vi "gRPC OOB Comm.vi"(6 "Main to gRPC":T2, 11 "Node in":refnum<class "ThermotronDriver.lvclass">) -> (1 "Update gRPC":bool, 3 "Node out":refnum<class "ThermotronDriver.lvclass">, 4 "gRPC to Main":T1)   [LabVIEW 2023, in "ThermotronDriver.lvlib" / "ThermotronDriver.lvclass"]
uses:
  ThermotronDriver.lvclass
  Type Defs/Main to gRPC.ctl
  Type Defs/gRPC to Main.ctl
  ThermotronDriver.lvclass/ThermotronDriver.ctl
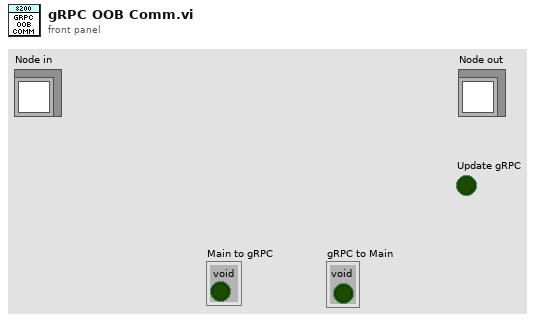
[diagram p1: front panel]
types:
  T1 = typedef "ThermotronDriver.lvlib/ThermotronDriver.lvclass/gRPC to Main.ctl" = cluster{"void":bool}
  T2 = typedef "ThermotronDriver.lvlib/ThermotronDriver.lvclass/Main to gRPC.ctl" = cluster{"void":bool}
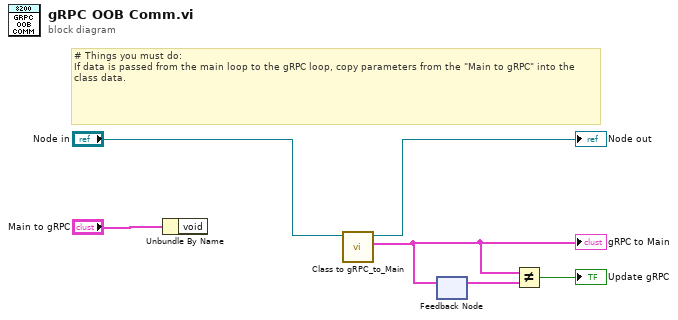
[diagram p0: block diagram]
diagram:
  # "# Things you must do:\nIf data is passed from the main loop to the gRPC loop, copy parameters from the \"Main to gRPC\" into the class data."
  n1 = Unbundle By Name("Main to gRPC") -> ()  [unwired: 1 out]
  n2 = call "Class to gRPC_to_Main.vi"("Timed Node in"="Node in") -> ("gRPC to Main"=w2:T1, "Timed Node out"=→"Node out":refnum<class "ThermotronDriver.lvclass">)  [unwired: 9 in]
  "gRPC to Main" <- w2
  n3 = feedback #1() -> (w6:T1)  [unwired: 1 in]
  n4 = feedback-in #1(w2) -> ()
  n5 = Not Equal?(x=w2, y=w6) -> (x != y?=→"Update gRPC":bool)
